vi "Initialize S3DK.vi"(8 "error in (no error)":errorcluster, 11 "Settings IN":T1={"State"=enum."Idle S3DK", "Settings"="", "S3DK"={"Signals"={"Phasor"=[], "Analog"=[], "Digital"=[]}}, "Tick"=0, "Online"=FALSE}) -> (0 "error out":errorcluster, 3 "Settings OUT":T1={"State"=enum."Idle S3DK", "Settings"="", "S3DK"={"Signals"={"Phasor"=[], "Analog"=[], "Digital"=[]}}, "Tick"=0, "Online"=FALSE})   [LabVIEW 2017, in "Acquisition.lvlib"]
doc: "Initialize the hardware references."
uses:
  Acquisition.lvlib
  Acquisition Settings.ctl
  Acquisition State.ctl
  <vilib>/S3DK/PMU Recorder Light/PMU Recorder Light.lvlib
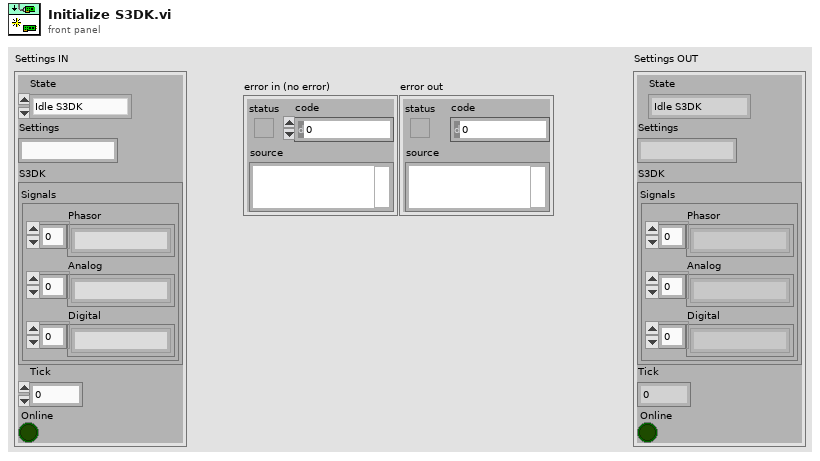
[diagram p1: front panel]
types:
  T1 = typedef "Acquisition.lvlib/Acquisition Settings.ctl" = cluster{"State":T2, "Settings":string, "S3DK":cluster{"Signals":cluster{"Phasor":string[], "Analog":string[], "Digital":string[]}}, "Tick":u32, "Online":bool}
  T2 = typedef "Acquisition.lvlib/Acquisition State.ctl" = enum16{"Idle", "Idle S3DK", "Acquiring S3DK", "Idle CSV", "Acquiring CSV"}
  T3 = enum16{"Run", "Startup", "Get Status", "Pause", "Continue", "Shutdown", "Abort", "Open Panel", "Close Panel"}
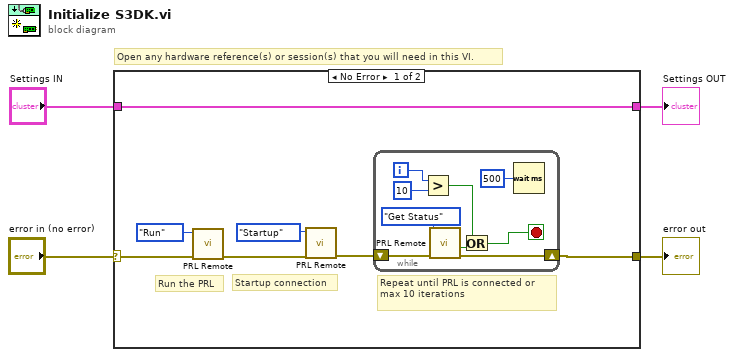
[diagram p0: block diagram]
diagram:
  # "Open any hardware reference(s) or session(s) that you will need in this VI."
  n1 = case shown="No Error" "error in (no error)" {
    selector: "error in (no error)" -> [w7 w21]
    tunnel: [w6 w21] -> w3
    tunnel: "Settings IN" -> [w11 w22]
    tunnel: [w11 w22] -> w1
    frame No Error {
      # "Repeat until PRL is connected or max 10 iterations"
      # "Startup connection"
      # "Run the PRL"
      n2 = call <vilib>:"PRL Remote.vi"("error in (no error)"=w7, "Action"=T3."Run") -> ("error out"=w9:errorcluster)  [unwired: 4 in, 5 out]
      n3 = call <vilib>:"PRL Remote.vi"("error in (no error)"=w9, "Action"=T3."Startup") -> ("error out"=w10:errorcluster)  [unwired: 4 in, 5 out]
      n4 = while {
        shift-right: [w13] -> w6
        shift-left: w10 -> [w12]
        i -> [w18]
        stop <- w19 stop-if-true
        n5 = Greater?(x=w18, y=10) -> (0:w16:bool)
        n6 = call <vilib>:"PRL Remote.vi"("error in (no error)"=w12, "Action"=T3."Get Status") -> ("error out"=w13:errorcluster, "Connected"=w15:bool)  [unwired: 4 in, 4 out]
        n7 = Or(x=w16, y=w15) -> (x .or. y?=w19:bool)
        n8 = Wait (ms)(milliseconds to wait=u32 500) -> ()  [unwired: 1 out]
      }
    }
    frame Error {
    }
  }
  "Settings OUT" <- w1
  "error out" <- w3
